vi "Read TDMS Wave.vi"(8 "error in (no error)":errorcluster, 9 "channel name(s) in":string, 10 "path":path, 11 "LVtoITX in":refnum<class "LVtoITX.lvclass">) -> (0 "error out":errorcluster, 2 "data":dbl[](array[numeric]), 3 "LVtoITX out":refnum<class "LVtoITX.lvclass">)   [LabVIEW 2016, in "LVtoITX.lvclass"]
uses:
  LVtoITX.lvclass
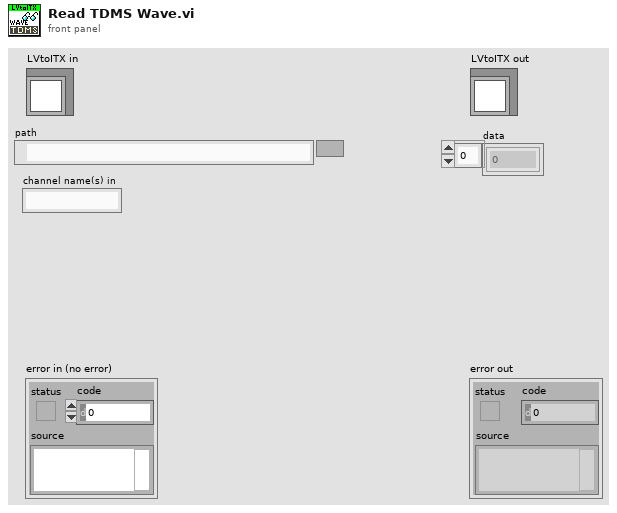
[diagram p1: front panel]
types:
  T1 = enum16{"open", "open or create", "create or replace", "create", "open (read-only)"}
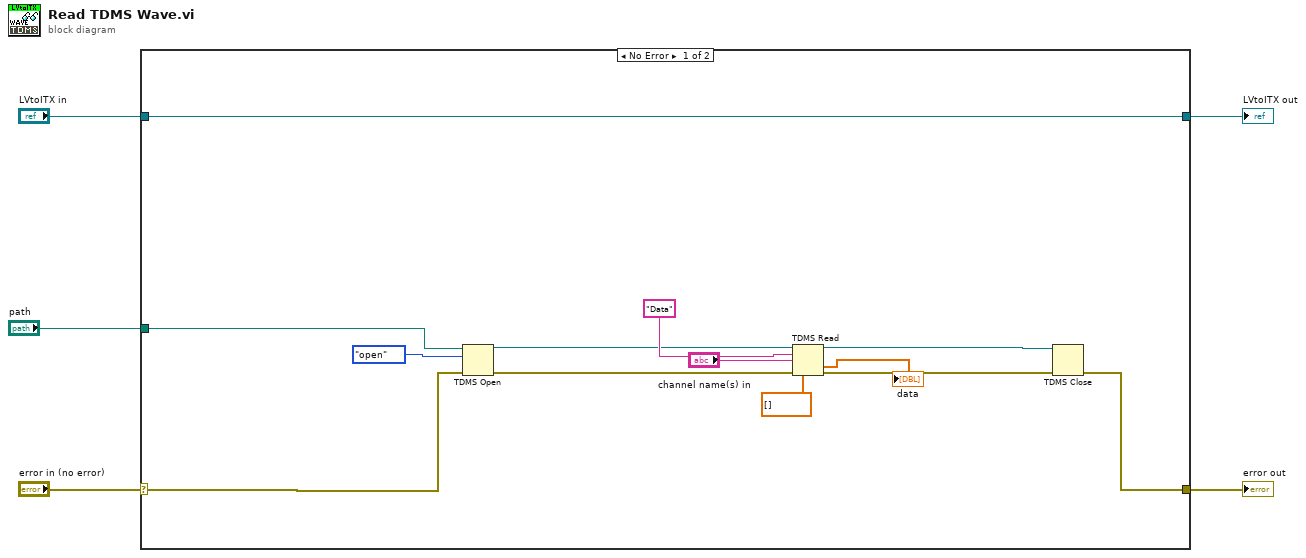
[diagram p0: block diagram]
diagram:
  n1 = case shown="No Error" "error in (no error)" {
    selector: "error in (no error)" -> [w14 w19]
    tunnel: [w17 w19] -> w2
    tunnel: [w7 w20] -> w3
    tunnel: "LVtoITX in" -> [w7 w20]
    tunnel: "path" -> [w13 _]
    frame No Error {
      n2 = TDMS Open(8:w14, 10:T1."open" ("operation (0:open)"), 11:w13) -> (0:w9:errorcluster, 3:w8:refnum<k34>)  [unwired: 4 in]
      n3 = TDMS Read(0:w8, 5:"Data" ("group name"), 7:"channel name(s) in", 11:w9, 12:dbl[] [] ("array type (2D Dbl)")) -> (4:w16:refnum<k34>, 10:→"data":dbl[], 15:w15:errorcluster)  [unwired: 3 in, 3 out]
      n4 = TDMS Close(8:w15, 11:w16) -> (0:w17:errorcluster)  [unwired: 1 out]
    }
    frame Error {
    }
  }
  "error out" <- w2
  "LVtoITX out" <- w3
